vi "LuaVIEW Get Function Documentation_srv.vi"(0 "function path":path, 7 "certificate":string) -> (4 "documentation":string, 8 "reentrant?":bool, 10 "synopsis":string, 15 "error out":errorcluster)   [LabVIEW 2012]
doc: "Returns the documentation, reentrancy, and synopsis of a server-side LuaVIEW function VI given a path to that VI. For this to work, the function must have been documented with the provided editor."
uses:
  clientsrv/typedefs/t_ClientSrv Access Levels.ctl
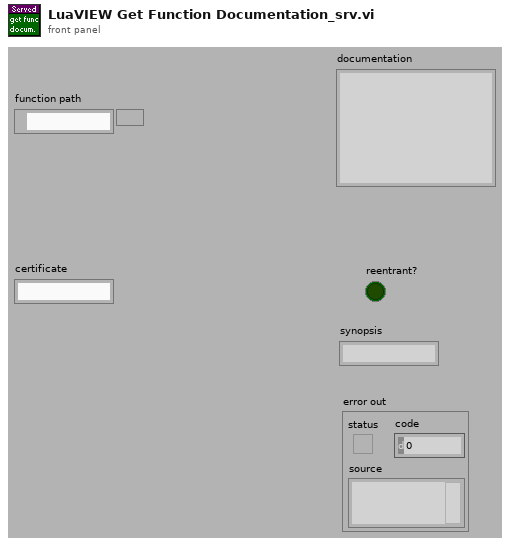
[diagram p1: front panel]
types:
  T1 = typedef "t_ClientSrv Access Levels.ctl" = enum16{"observer", "operator", "local"}
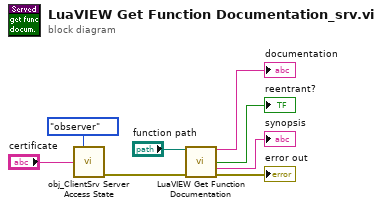
[diagram p0: block diagram]
diagram:
  n1 = call "obj_ClientSrv Server Access State.vi"("access level"=t_ClientSrv_Access_Levels."observer", "certificate in"="certificate") -> ("error out"=w6:errorcluster)  [unwired: 11 in, 2 out]
  n2 = call "LuaVIEW Get Function Documentation.vi"("function path"="function path", "error in (no error)"=w6) -> ("documentation"=→"documentation":string, "reentrant?"=→"reentrant?":bool, "synopsis"=→"synopsis":string, "error out"=→"error out":errorcluster)  [unwired: 10 in]
